vi "EPS-Configure Operation Value.vi"(8 "error in":errorcluster, 9 "Values":dbl format="%#.3g", 10 "Value Type":T1, 11 "EPS Setting In":T2) -> (0 "error out":errorcluster, 3 "EPS Setting Out":T2)   [LabVIEW 2018]
uses:
  Data Def/EPS-Setting.ctl
  Data Def/EPS-Value Type.ctl
  Data Def/EPS-Access Mode.ctl
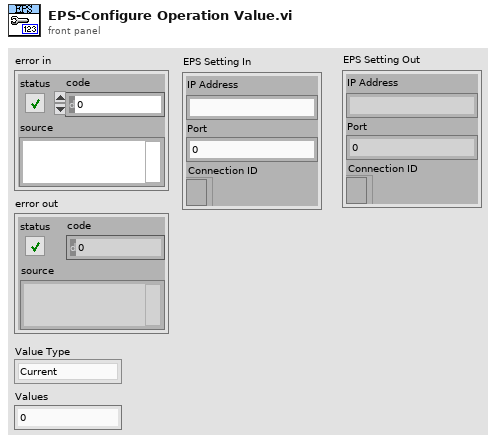
[diagram p1: front panel]
types:
  T1 = typedef "EPS-Value Type.ctl" = enum16{"Current", "Vlotage", "Power"}
  T2 = typedef "EPS-Setting.ctl" = cluster{"IP Address":string, "Port":u16, "Connection ID":refnum<k5>}
  T3 = typedef "EPS-Access Mode.ctl" = enum16{"Read", "Write"}
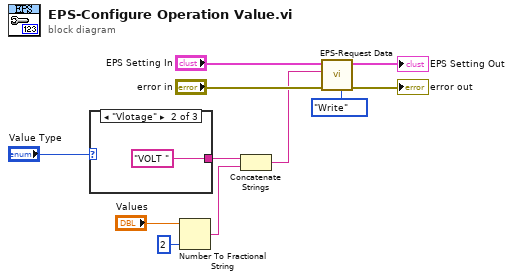
[diagram p0: block diagram]
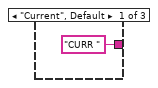
[diagram p2: hidden frame]
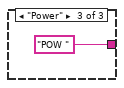
[diagram p3: hidden frame]
diagram:
  n1 = case shown="\"Vlotage\"" "Value Type" {
    tunnel: ["CURR " "VOLT " "POW "] -> w3
    frame "Current", Default {
    }
    frame "Vlotage" {
    }
    frame "Power" {
    }
  }
  n2 = Number To Fractional String(number="Values", precision (6)=i16 2) -> (F-format string=w2:string)  [unwired: 2 in]
  n3 = Concatenate Strings(w3, w2) -> (w1:string)
  n4 = call "EPS-Request Data.vi"("Access Mode"=EPS-Access_Mode."Write", "error in"="error in", "Requst Data"=w1, "EPS Setting In"="EPS Setting In") -> ("error out"=→"error out":errorcluster, "EPS Setting Out"=→"EPS Setting Out":T2)  [unwired: 5 in, 1 out]
